vi "CodeToStr.vi"(11 "Name in":string="Name in") -> (3 "Name out":string)   [LabVIEW 2019]
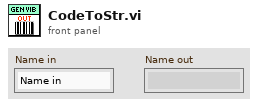
[diagram p1: front panel]
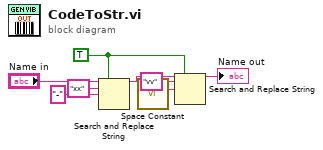
[diagram p0: block diagram]
diagram:
  w5 = TRUE ("replace all? (F)")
  n1 = Search and Replace String(replace all?=w5, input string="Name in", search string="xx", replace string="-" ("replace string (\"\")")) -> (result string=w4:string)  [unwired: 4 in, 3 out]
  n2 = call <vilib>:"Space Constant.vi"() -> ("String"=w3:string)
  n3 = Search and Replace String(replace all?=w5, input string=w4, search string="vv" ("replace string (\"\")"), replace string=w3) -> (result string=→"Name out":string)  [unwired: 4 in, 3 out]
